vi "save.indices.vi"(8 "error in (no error)":errorcluster, 11 "manager_daemon in":refnum<class "manager_daemon.lvclass">) -> (0 "error out":errorcluster, 3 "manager_daemon out":refnum<class "manager_daemon.lvclass">)   [LabVIEW 2024, in "manager_daemon.lvclass"]
uses:
  manager_daemon.lvclass
  manager_daemon.lvclass/manager_daemon.ctl
  7b70191b-b604-4134-9c84-a7eca9edbca5.vi
  8ee442e6-0590-49e2-b6e3-9d7b8bb6845c.vi
  5a9fdcdc-2837-4a82-9f52-23d004c71c28.vi
  4c834036-f134-4293-ba3f-71b30b6c426d.vi
  858a4df7-9059-4d7a-91f7-1fe4ab9969b3.vi
  3b8794f8-cd8f-4bab-ab67-d464a98a7a60.vi
  0fbe7c90-43c9-43a5-9013-a6c576da65e3.vi
  27209167-718f-44ea-8cf2-7e7bccf769dc.vi
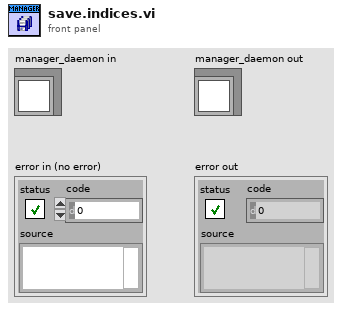
[diagram p1: front panel]
types:
  T1 = typedef "manager_daemon.lvclass/VolumeData--cluster.ctl" = cluster{"name":string, "sortable_name":string, "aliases":string[], "description":string, "site_detail_url":string, "count_of_issues":i32, "start_year":i32, "publisher_id":i32, "issue_ids":i32[], "date_last_updated":timestamp, "volume":i32, "cv_id":string, "volume type":T2, "source_path":path}
  T2 = typedef "CV_Shared_Library.lvlib/volume.type--enum.ctl" = enum16{"Ongoing", "Limited Series", "Annual", "One Shot", "Reprint/Document", "Star Comics", "Epic Comics"}
  T3 = typedef "manager_daemon.lvclass/IssueData--clustrer.ctl" = cluster{"cover_date":timestamp, "cv_id":string, "name":string, "sortable_name":string, "issue_number":string, "deck":string, "description":string, "id":i32, "store_date":timestamp, "date_last_updated":timestamp, "site_detail_url":string, "cover_url":string, "source_path":path, "character map":map{i32, string}, "concept map":map{i32, string}, "storyArc map":map{i32, string}, "team map":map{i32, string}, "creator map":map{i32, cluster{"name":string, "role":string}}}
  T4 = typedef "manager_daemon.lvclass/sub-map--map.ctl" = map{string, T5}
  T5 = typedef "manager_daemon.lvclass/SubData--cluster.ctl" = cluster{"id":i32, "issues":set{i32}}
  T6 = map{string, set{cluster{"id":i32, "role":string}}}
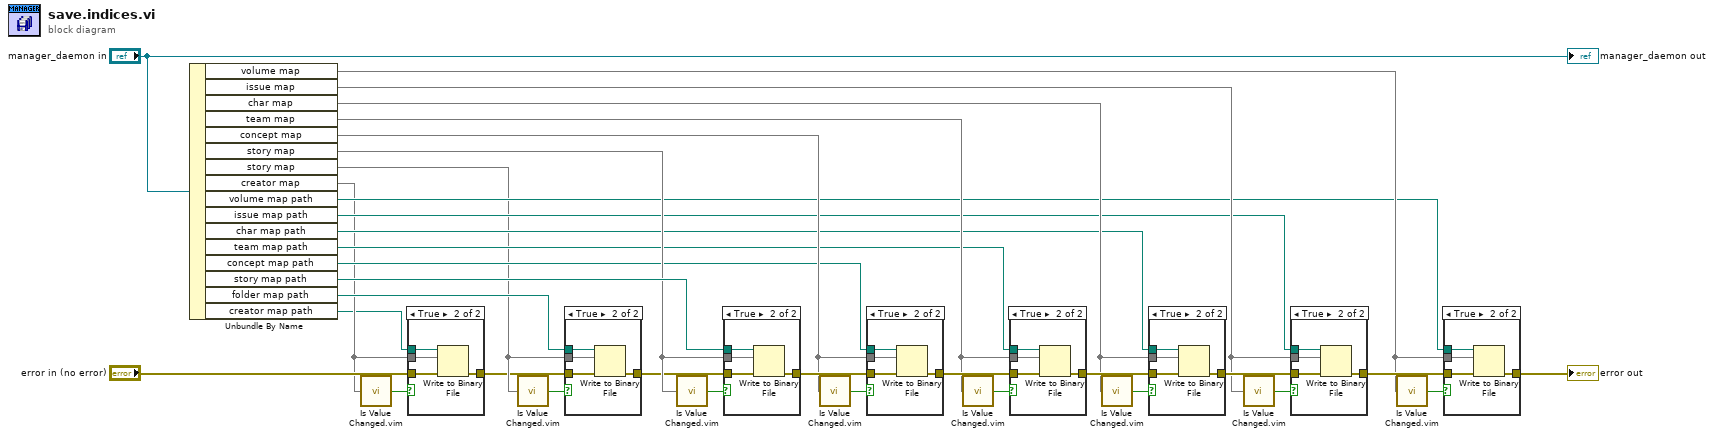
[diagram p0: block diagram]
diagram:
  n1 = Unbundle By Name("manager_daemon in") -> ("volume map"=w15:map{i32, T1}, "issue map"=w16:map{i32, T3}, "char map"=w17:T4, "team map"=w18:T4, "concept map"=w19:T4, "story map"=w32:T4, "story map"=w7:T4, "creator map"=w2:T6, "volume map path"=w10:path, "issue map path"=w11:path, "char map path"=w12:path, "team map path"=w13:path, "concept map path"=w14:path, "story map path"=w33:path, "folder map path"=w8:path, "creator map path"=w1:path)
  n2 = call "Is Value Changed.vim"("value"=w2) -> ("changed or first call?"=w3:bool)
  n3 = case shown="True" w3 {
    tunnel: "error in (no error)" -> [w35 w39]
    tunnel: [w35 w38] -> w5
    tunnel: w1 -> [_ w37]
    tunnel: w2 -> [_ w36]
    frame False {
    }
    frame True {
      n4 = Write to Binary File(file (use dialog)=w37, data=w36, error in=w39) -> (error out=w38:errorcluster)  [unwired: 3 in, 2 out]
    }
  }
  n5 = call "Is Value Changed.vim"("value"=w7) -> ("changed or first call?"=w6:bool)
  n6 = case shown="True" w6 {
    tunnel: w5 -> [w40 w44]
    tunnel: [w40 w43] -> w9
    tunnel: w8 -> [_ w42]
    tunnel: w7 -> [_ w41]
    frame False {
    }
    frame True {
      n7 = Write to Binary File(file (use dialog)=w42, data=w41, error in=w44) -> (error out=w43:errorcluster)  [unwired: 3 in, 2 out]
    }
  }
  n8 = call "Is Value Changed.vim"("value"=w32) -> ("changed or first call?"=w31:bool)
  n9 = case shown="True" w31 {
    tunnel: w9 -> [w45 w49]
    tunnel: [w45 w48] -> w30
    tunnel: w33 -> [_ w47]
    tunnel: w32 -> [_ w46]
    frame False {
    }
    frame True {
      n10 = Write to Binary File(file (use dialog)=w47, data=w46, error in=w49) -> (error out=w48:errorcluster)  [unwired: 3 in, 2 out]
    }
  }
  n11 = call "Is Value Changed.vim"("value"=w19) -> ("changed or first call?"=w24:bool)
  n12 = case shown="True" w24 {
    tunnel: w30 -> [w50 w54]
    tunnel: [w50 w53] -> w29
    tunnel: w14 -> [_ w52]
    tunnel: w19 -> [_ w51]
    frame False {
    }
    frame True {
      n13 = Write to Binary File(file (use dialog)=w52, data=w51, error in=w54) -> (error out=w53:errorcluster)  [unwired: 3 in, 2 out]
    }
  }
  n14 = call "Is Value Changed.vim"("value"=w18) -> ("changed or first call?"=w23:bool)
  n15 = case shown="True" w23 {
    tunnel: w29 -> [w55 w59]
    tunnel: [w55 w58] -> w28
    tunnel: w13 -> [_ w57]
    tunnel: w18 -> [_ w56]
    frame False {
    }
    frame True {
      n16 = Write to Binary File(file (use dialog)=w57, data=w56, error in=w59) -> (error out=w58:errorcluster)  [unwired: 3 in, 2 out]
    }
  }
  n17 = call "Is Value Changed.vim"("value"=w17) -> ("changed or first call?"=w22:bool)
  n18 = case shown="True" w22 {
    tunnel: w28 -> [w60 w64]
    tunnel: [w60 w63] -> w27
    tunnel: w12 -> [_ w62]
    tunnel: w17 -> [_ w61]
    frame False {
    }
    frame True {
      n19 = Write to Binary File(file (use dialog)=w62, data=w61, error in=w64) -> (error out=w63:errorcluster)  [unwired: 3 in, 2 out]
    }
  }
  n20 = call "Is Value Changed.vim"("value"=w16) -> ("changed or first call?"=w21:bool)
  n21 = case shown="True" w21 {
    tunnel: w27 -> [w65 w69]
    tunnel: [w65 w68] -> w26
    tunnel: w11 -> [_ w67]
    tunnel: w16 -> [_ w66]
    frame False {
    }
    frame True {
      n22 = Write to Binary File(file (use dialog)=w67, data=w66, error in=w69) -> (error out=w68:errorcluster)  [unwired: 3 in, 2 out]
    }
  }
  n23 = call "Is Value Changed.vim"("value"=w15) -> ("changed or first call?"=w20:bool)
  n24 = case shown="True" w20 {
    tunnel: w26 -> [w70 w74]
    tunnel: [w70 w73] -> w25
    tunnel: w10 -> [_ w72]
    tunnel: w15 -> [_ w71]
    frame False {
    }
    frame True {
      n25 = Write to Binary File(file (use dialog)=w72, data=w71, error in=w74) -> (error out=w73:errorcluster)  [unwired: 3 in, 2 out]
    }
  }
  "error out" <- w25
  "manager_daemon out" <- "manager_daemon in"
